vi "FindSubimage.vi"(8 "Scale factor (1)":dbl=1.0 format="%#_13g", 9 "ROI (left top right bottom)":u32[](array[numeric])=[0, 0, 5000, 5000], 10 "RGB Template":T1, 11 "RGB Image":T1) -> (3 "Locations (left, top)":dbl[](array[numeric]))   [LabVIEW 2014]
uses:
  <vilib>/vision/Image Controls.llb/IMAQ Image.ctl
  CalculateSSDImages.vi
  2D Array/Search 2D Array (Bool).vi
  <vilib>/vision/NI_Vision_Development_Module.lvlib
  <vilib>/addons/Machine Learning/NILabs_MLT.lvlib
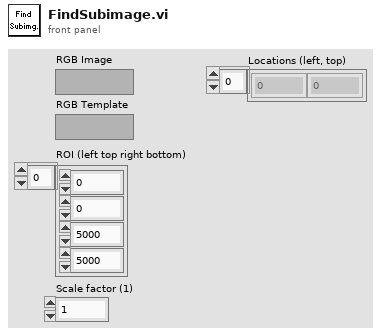
[diagram p1: front panel]
types:
  T1 = typedef "IMAQ Image.ctl" = refnum<image>
  T2 = typedef "Image Type" = u32
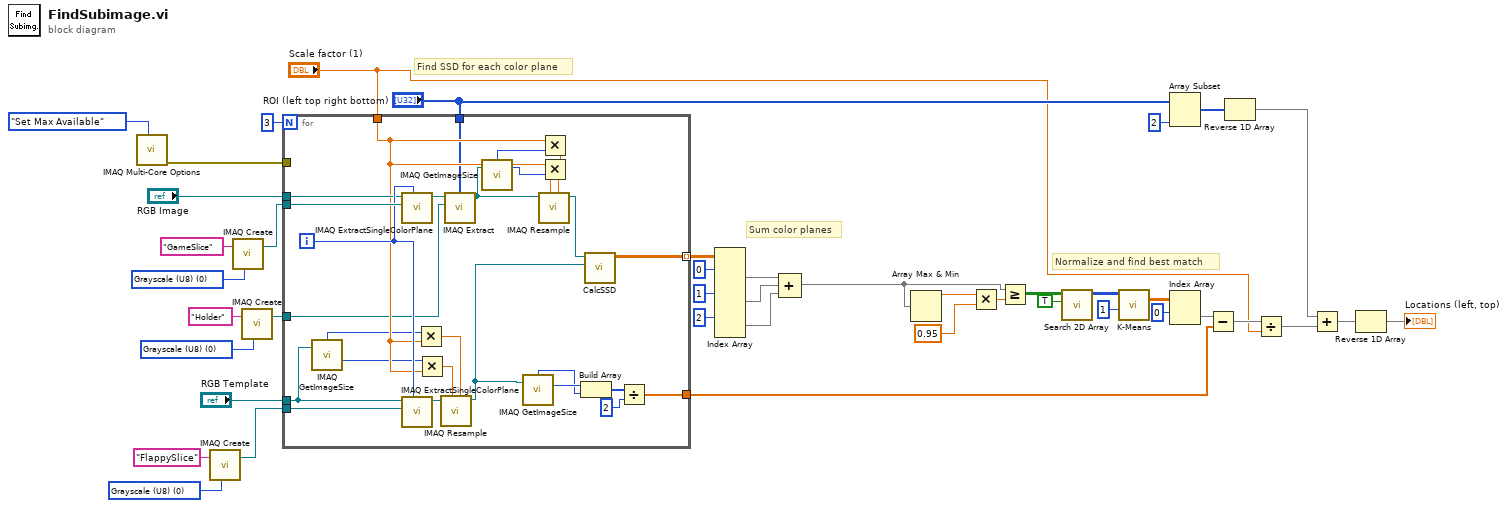
[diagram p0: block diagram]
diagram:
  w11 = T2 0 items=["Grayscale (U8)", "Grayscale (I16)", "Grayscale (SGL)", "Complex (CSG)", "RGB (U32)", "HSL (U32)", "RGB (U64)", "Grayscale (U16)"] ("Image Type")
  w36 = T2 0 items=["Grayscale (U8)", "Grayscale (I16)", "Grayscale (SGL)", "Complex (CSG)", "RGB (U32)", "HSL (U32)", "RGB (U64)", "Grayscale (U16)"] ("Image Type")
  w39 = T2 0 items=["Grayscale (U8)", "Grayscale (I16)", "Grayscale (SGL)", "Complex (CSG)", "RGB (U32)", "HSL (U32)", "RGB (U64)", "Grayscale (U16)"] ("Image Type")
  # "Sum color planes"
  # "Find SSD for each color plane"
  # "Normalize and find best match"
  n1 = call "IMAQ Multi-Core Options"("Get/Set Number of Cores (Get)"=enum32{"Get", "Set", "Set Max Available"}."Set Max Available") -> ("error out"=w15:errorcluster)  [unwired: 9 in, 1 out]
  n2 = call "IMAQ Create"("Image Name"="FlappySlice", "Image Type"=w39) -> ("New Image"=w38:T1)  [unwired: 3 in, 1 out]
  n3 = call "IMAQ Create"("Image Name"="GameSlice", "Image Type"=w36) -> ("New Image"=w35:T1)  [unwired: 3 in, 1 out]
  n4 = call "IMAQ Create"("Image Name"="Holder", "Image Type"=w11) -> ("New Image"=w9:T1)  [unwired: 3 in, 1 out]
  n5 = for {
    N: 3 -> [_]
    tunnel: w38 -> [w69]
    tunnel: w35 -> [w68]
    tunnel: "RGB Template" -> [w60]
    tunnel: "RGB Image" -> [w65]
    tunnel: [w67] -> w34 mode=indexing
    tunnel: "ROI (left top right bottom)" -> [w51]
    tunnel: w15 -> [_]
    tunnel: "Scale factor (1)" -> [w57]
    tunnel: [w52] -> w7
    tunnel: w9 -> [w49]
    i -> [w66]
    n6 = call "IMAQ GetImageSize"("Image"=w60) -> ("Y Resolution"=w55:i32, "X Resolution"=w54:i32)  [unwired: 3 in, 1 out]
    n7 = call "IMAQ ExtractSingleColorPlane"("Color Plane"=w66, "Image Dst"=w68, "Image Src"=w65) -> ("Image Dst Out"=w50:T1)  [unwired: 7 in, 1 out]
    n8 = call "IMAQ ExtractSingleColorPlane"("Color Plane"=w66, "Image Dst"=w69, "Image Src"=w60) -> ("Image Dst Out"=w59:T1)  [unwired: 7 in, 1 out]
    n9 = Multiply(x=w54, y=w57) -> (x*y=w58:dbl)
    n10 = Multiply(x=w55, y=w57) -> (x*y=w56:dbl)
    n11 = call "IMAQ Resample"("X Resolution"=w58, "Y Resolution"=w56, "Image Src"=w59) -> ("Image Dst Out"=w46:T1)  [unwired: 7 in, 1 out]
    n12 = call "IMAQ Extract"("Optional Rectangle"=w51, "Image Dst"=w49, "Image Src"=w50) -> ("Image Dst Out"=w48:T1)  [unwired: 7 in, 1 out]
    n13 = call "IMAQ GetImageSize"("Image"=w48) -> ("Y Resolution"=w64:i32, "X Resolution"=w63:i32)  [unwired: 3 in, 1 out]
    n14 = call "IMAQ GetImageSize"("Image"=w46) -> ("Y Resolution"=w44:i32, "X Resolution"=w43:i32)  [unwired: 3 in, 1 out]
    n15 = Multiply(x=w57, y=w63) -> (x*y=w61:dbl)
    n16 = Multiply(x=w57, y=w64) -> (x*y=w62:dbl)
    n17 = call "IMAQ Resample"("X Resolution"=w61, "Y Resolution"=w62, "Image Src"=w48) -> ("Image Dst Out"=w47:T1)  [unwired: 7 in, 1 out]
    n18 = Build Array(w44, w43) -> (w45:i32[])
    n19 = call-poly "CalcSSD.vi"("Template"=w46, "Image"=w47) -> ("SSD"=w67:dbl[][])  [unwired: 9 in]
    n20 = Divide(x=w45, y=2 ("X Resolution")) -> (x/y=w52:dbl[])
  }
  n21 = Index Array(array=w34, index (dim 0) #1=0 ("index (page)"), index (dim 0) #2=1 ("index (page)"), index (dim 0) #3=2 ("index (page)")) -> (element #1=w32:dbl[][], element #2=w18:dbl[][], element #3=w17:dbl[][])  [unwired: 6 in]
  n22 = Compound Arithmetic op=ADD(w32, w18, w17) -> (w12:dbl[][])
  n23 = Array Max & Min(array=w12) -> (max value=w42:dbl)  [unwired: 3 out]
  n24 = Multiply(x=w42, y=0.95 ("SSD Threshold (0.95)")) -> (x*y=w41:dbl)
  n25 = Greater Or Equal?(x=w12, y=w41) -> (x >= y?=w13:bool[][])
  n26 = call-poly "Search 2D Array.vi"("Element"=TRUE, "Array"=w13) -> ("Locations"=w29:i32[][])  [unwired: 9 in]
  n27 = call <vilib>:"K-Means.vi"("# of classes"=1, "Data samples"=w29) -> ("Centroids"=w26:dbl[][])  [unwired: 7 in, 2 out]
  n28 = Array Subset(array="ROI (left top right bottom)", length=2) -> (w5:u32[])  [unwired: 1 in]
  n29 = Index Array(array=w26, index (row)=0) -> (element=w8:dbl[])  [unwired: 1 in]
  n30 = Subtract(x=w8, y=w7) -> (x-y=w6:dbl[])
  n31 = Reverse 1D Array(array=w5) -> (reversed array=w4:u32[])
  n32 = Divide(x=w6, y="Scale factor (1)") -> (x/y=w14:dbl[])
  n33 = Add(x=w4, y=w14) -> (x+y=w2:dbl[])
  n34 = Reverse 1D Array(array=w2) -> (reversed array=→"Locations (left, top)":dbl[])
